vi "Write Config Section.vi"(8 "error in (no error)":errorcluster, 10 "Config Section":string, 11 "Configurable Device in":refnum<class "Configurable Device.lvclass">) -> (0 "error out":errorcluster, 3 "Configurable Device out":refnum<class "Configurable Device.lvclass">)   [LabVIEW 2014, in "Device.lvlib" / "Configurable Device.lvclass"]
uses:
  Configurable Device.lvclass
  Configurable Device.lvclass/Configurable Device.ctl
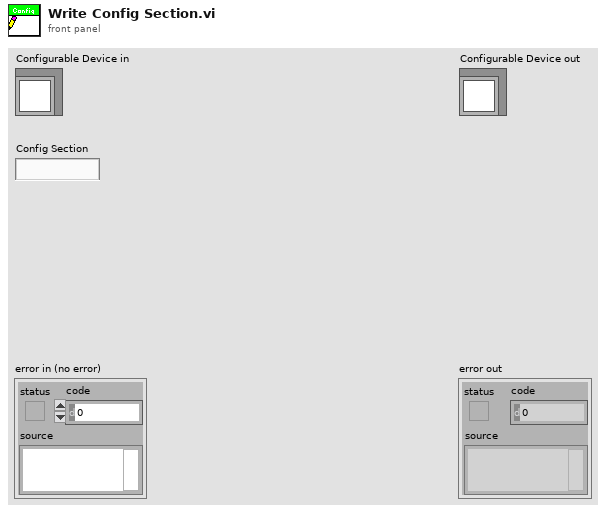
[diagram p1: front panel]
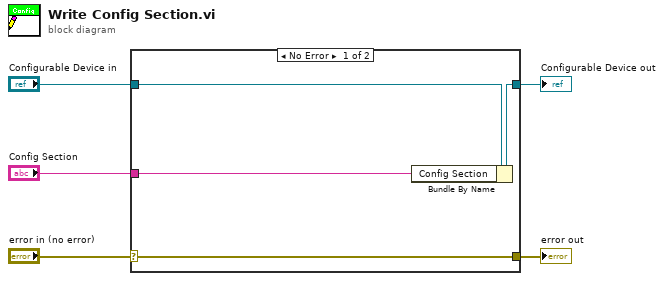
[diagram p0: block diagram]
diagram:
  n1 = case shown="No Error" "error in (no error)" {
    selector: "error in (no error)" -> [w9 w10]
    tunnel: [w9 w10] -> w4
    tunnel: [w7 w11] -> w2
    tunnel: "Configurable Device in" -> [w8 w11]
    tunnel: "Config Section" -> [w6 _]
    frame No Error {
      n2 = Bundle By Name(cluster=w8, "Config Section"=w6) -> (w7:refnum<class "Configurable Device.lvclass">)
    }
    frame Error {
    }
  }
  "error out" <- w4
  "Configurable Device out" <- w2
